vi "ReadHooverOverInfo.vi"(8 "error in (no error)":errorcluster, 11 "Parameter in":refnum<class "Parameter.lvclass">) -> (0 "error out":errorcluster, 2 "HooverOverInfo":string, 3 "Parameter out":refnum<class "Parameter.lvclass">)   [LabVIEW 2023, in "Easy.SequenceManagerLabVIEW.lvlib" / "Parameter.lvclass"]
uses:
  Parameter.lvclass
  Parameter.lvclass/Parameter.ctl
panel:
  # "Connector Pane"
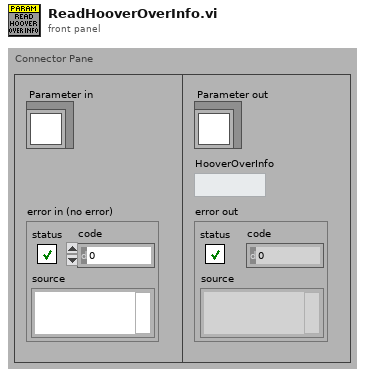
[diagram p1: front panel]
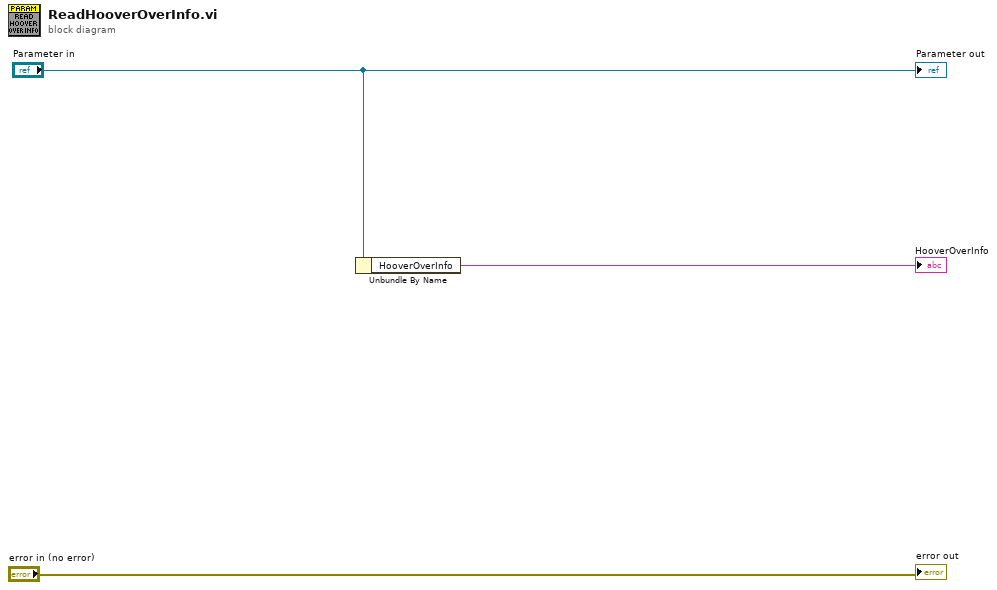
[diagram p0: block diagram]
diagram:
  n1 = Unbundle By Name("Parameter in") -> ("HooverOverInfo"=→"HooverOverInfo":string)
  "error out" <- "error in (no error)"
  "Parameter out" <- "Parameter in"
